vi "DriveTeleop.vi"(11 "JoystickData":T1) -> ()   [LabVIEW 2018]
uses:
  Framework/Robot Global Data.vi
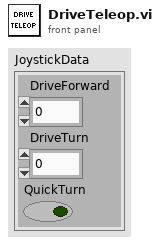
[diagram p1: front panel]
types:
  T1 = cluster{"DriveForward":dbl, "DriveTurn":dbl, "QuickTurn":bool}
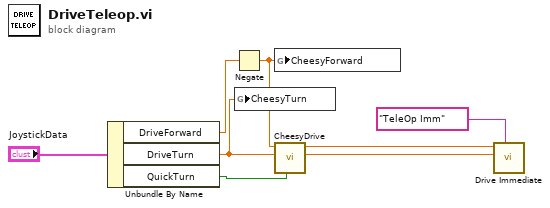
[diagram p0: block diagram]
diagram:
  n1 = Unbundle By Name("JoystickData") -> ("DriveForward"=w4:dbl, "DriveTurn"=w3:dbl, "QuickTurn"=w2:bool)
  n2 = Negate(x=w4) -> (-x=w5:dbl)
  n3 = global write "Robot Global Data.vi" "CheesyTurn"(w3) -> ()
  n4 = global write "Robot Global Data.vi" "CheesyForward"(w5) -> ()
  n5 = call "CheesyDrive.vi"("Quickturn"=w2, "Wheel"=w3, "Throttle"=w5) -> ("Right PWM"=w7:dbl, "Left PWM"=w8:dbl)  [unwired: 7 in]
  n6 = call "Drive Immediate.vi"("Description"="TeleOp Imm", "Right Setpoint"=w7, "Left Setpoint"=w8) -> ()  [unwired: 8 in, 1 out]
